vi "Write Source.vi"(8 "error in (no error)":errorcluster, 10 "Source":path, 11 "Job.SingleFileCopy in":refnum<class "Job.SingleFileCopy.lvclass">) -> (0 "error out":errorcluster, 3 "Job.SingleFileCopy out":refnum<class "Job.SingleFileCopy.lvclass">)   [LabVIEW 2013, in "Job.SingleFileCopy.lvclass"]
uses:
  Job.SingleFileCopy.lvclass
  Job.SingleFileCopy.lvclass/Job.SingleFileCopy.ctl
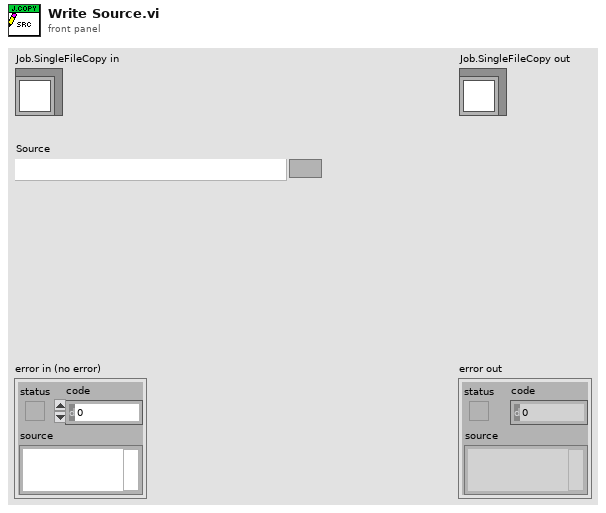
[diagram p1: front panel]
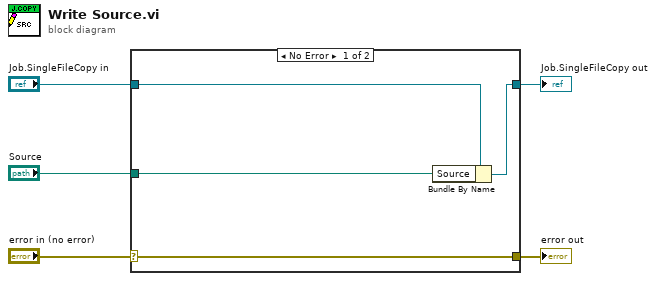
[diagram p0: block diagram]
diagram:
  n1 = case shown="No Error" "error in (no error)" {
    selector: "error in (no error)" -> [w9 w10]
    tunnel: [w9 w10] -> w4
    tunnel: [w7 w11] -> w2
    tunnel: "Job.SingleFileCopy in" -> [w8 w11]
    tunnel: "Source" -> [w6 _]
    frame No Error {
      n2 = Bundle By Name(cluster=w8, "Source"=w6) -> (w7:refnum<class "Job.SingleFileCopy.lvclass">)
    }
    frame Error {
    }
  }
  "error out" <- w4
  "Job.SingleFileCopy out" <- w2
